vi "GetGXMLCfgThrmcpl.vi"(8 "error in (no error)":errorcluster, 11 "Thermocouple in":refnum<class "Thermocouple.lvclass">) -> (0 "error out":errorcluster, 2 "ThrmcplChanCfg":T1, 3 "Thermocouple out":refnum<class "Thermocouple.lvclass">)   [LabVIEW 2018, in "Measurement Channels.lvlib" / "Thermocouple.lvclass"]
uses:
  Thermocouple.lvclass
  ThrmcplProps_TD.ctl
  Thermocouple.lvclass/Thermocouple.ctl
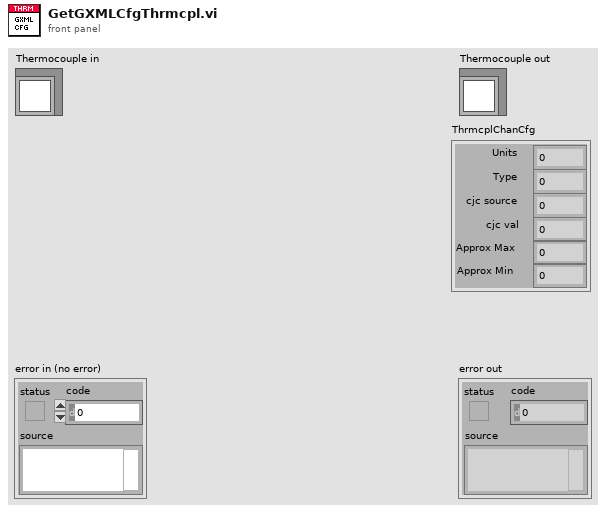
[diagram p1: front panel]
types:
  T1 = typedef "Measurement Channels.lvlib/Thermocouple.lvclass/ThrmcplProps_TD.ctl" = cluster{"Units":u16, "Type":u16, "cjc source":u16, "cjc val":dbl, "Approx Max":dbl, "Approx Min":dbl}
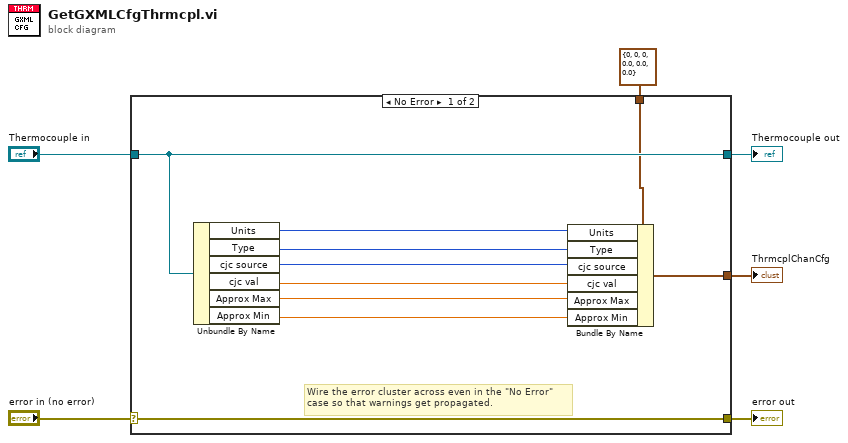
[diagram p0: block diagram]
diagram:
  n1 = case shown="No Error" "error in (no error)" {
    selector: "error in (no error)" -> [w16 w19]
    tunnel: [w16 w19] -> w5
    tunnel: [w15 w18] -> w3
    tunnel: "Thermocouple in" -> [w15 w18]
    tunnel: T1 {"Units"=0, "Type"=0, "cjc source"=0, "cjc val"=0.0, "Approx Max"=0.0, "Approx Min"=0.0} ("ThrmcplChanCfg") -> [w13 w17]
    tunnel: [w7 w17] -> w1
    frame No Error {
      # "Wire the error cluster across even in the \"No Error\"\ncase so that warnings get propagated."
      n2 = Unbundle By Name(w15) -> ("Units"=w14:u16, "Type"=w12:u16, "cjc source"=w11:u16, "cjc val"=w10:dbl, "Approx Max"=w9:dbl, "Approx Min"=w8:dbl)
      n3 = Bundle By Name(cluster=w13, "Units"=w14, "Type"=w12, "cjc source"=w11, "cjc val"=w10, "Approx Max"=w9, "Approx Min"=w8) -> (w7:T1)
    }
    frame Error {
    }
  }
  "error out" <- w5
  "Thermocouple out" <- w3
  "ThrmcplChanCfg" <- w1
